vi "oa_Check Tach Pulses Data for Waveform Reference (N Channels).vi"(7 "reset? (True)":bool=TRUE, 8 "error in (no error)":errorcluster, 9 "interpolated pulse positions":dbl[](array[numeric]) format="%.2f", 10 "speed profile":T1 {"speed [RPM]" format="%.2f"; "time [s]" format="%.2f"}, 11 "even angle signals":cluster{"r0":dbl, "dr":dbl, "Y":dbl[]}[](array[cluster]) {"r0" format="%.2p"; "dr" format="%.2p"; "Y" format="%.2f"}) -> (0 "error out":errorcluster, 1 "interpolated pulse positions out":dbl[](array[numeric]) format="%.2f", 2 "speed profile out":T1 {"speed [RPM]" format="%.2f"; "time [s]" format="%.2f"}, 3 "even angle signals":cluster{"r0":dbl, "dr":dbl, "Y":dbl[]}[](array[cluster]) {"r0" format="%.2p"; "dr" format="%.2p"; "Y" format="%.2f"}, 5 "reset":bool)   [LabVIEW 2017]
uses:
  <vilib>/addons/Sound and Vibration/Order Analysis/Tach Process/SubVIs/speed profile.ctl
  <vilib>/addons/Sound and Vibration/Order Analysis/Tach Process/SoundVib_TachProcess.lvlib
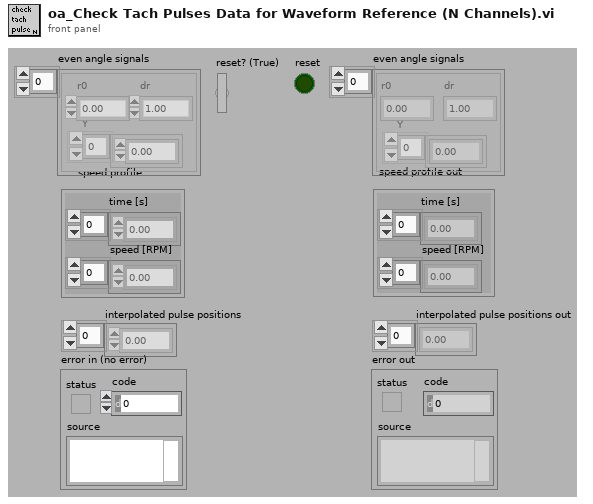
[diagram p1: front panel]
types:
  T1 = typedef "SoundVib_TachProcess.lvlib/speed profile.ctl" = cluster{"time [s]":dbl[], "speed [RPM]":dbl[]}
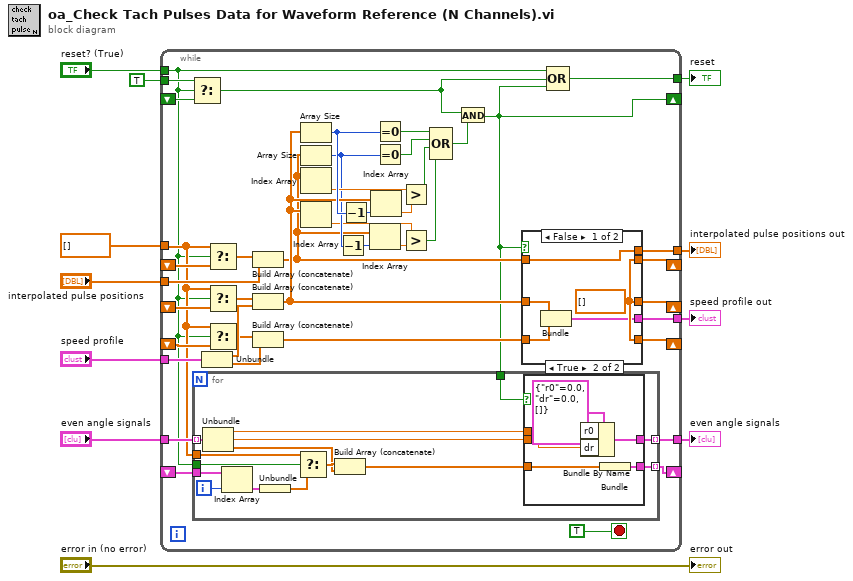
[diagram p0: block diagram]
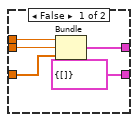
[diagram p2: hidden frame]
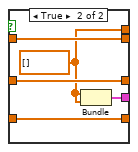
[diagram p3: hidden frame]
diagram:
  n1 = while {
    tunnel: "reset? (True)" -> [w15]
    shift-right: [w13] -> _
    shift-left: _ -> [w53]
    tunnel: "interpolated pulse positions" -> [w48]
    tunnel: "speed profile" -> [w52]
    tunnel: "even angle signals" -> [w51]
    shift-right: [w20] -> _
    shift-left: _ -> [w19]
    tunnel: dbl[] [] ("Y") -> [w18]
    shift-right: [w47] -> _
    shift-left: _ -> [w50]
    tunnel: [w46] -> w4
    shift-right: [w43] -> _
    shift-left: _ -> [w45]
    shift-right: [w38] -> _
    shift-left: _ -> [w40]
    tunnel: [w36] -> w7
    tunnel: TRUE -> [w35]
    tunnel: [w17] -> w2
    tunnel: [w12] -> w1
    stop <- TRUE stop-if-true
    n2 = Select(t=w35, s=w15, f=w53) -> (s? t:f=w14:bool)
    n3 = Unbundle(w52) -> ("time [s]"=w44:dbl[], "speed [RPM]"=w39:dbl[])
    n4 = Select(t=w18, s=w15, f=w50) -> (s? t:f=w49:dbl[])
    n5 = Select(t=w18, s=w15, f=w45) -> (s? t:f=w41:dbl[])
    n6 = Select(t=w18, s=w15, f=w40) -> (s? t:f=w42:dbl[])
    n7 = Build Array (concatenate)(w49, w48) -> (w28:dbl[])
    n8 = Build Array (concatenate)(w41, w44) -> (w31:dbl[])
    n9 = Build Array (concatenate)(w42, w39) -> (w37:dbl[])
    n10 = Array Size(array=w31) -> (size(s)=w34:i32)
    n11 = Array Size(array=w28) -> (size(s)=w29:i32)
    n12 = Index Array(array=w28) -> (element=w33:dbl)  [unwired: 1 in]
    n13 = Index Array(array=w31) -> (element=w25:dbl)  [unwired: 1 in]
    n14 = Decrement(x=w29) -> (x-1=w27:i32)
    n15 = Decrement(x=w34) -> (x-1=w30:i32)
    n16 = Index Array(array=w28, index=w27) -> (element=w26:dbl)
    n17 = Index Array(array=w31, index=w30) -> (element=w32:dbl)
    n18 = Equal To 0?(x=w34) -> (x = 0?=w24:bool)
    n19 = Equal To 0?(x=w29) -> (x = 0?=w23:bool)
    n20 = Greater?(x=w33, y=w32) -> (0:w22:bool)
    n21 = Greater?(x=w25, y=w26) -> (0:w21:bool)
    n22 = Compound Arithmetic op=OR(w24, w23, w22, w21) -> (w16:bool)
    n23 = And(x=w14, y=w16) -> (x .and. y?=w13:bool)
    n24 = for {
      tunnel: w19 -> [w60]
      tunnel: w51 -> [w69] mode=indexing
      tunnel: w15 -> [w67]
      tunnel: w13 -> [w66]
      tunnel: [w62] -> w20 mode=indexing
      tunnel: w18 -> [w61]
      tunnel: [w55] -> w17 mode=indexing
      i -> [w58]
      n25 = Unbundle(w69) -> ("r0"=w65:dbl, "dr"=w64:dbl, "Y"=w59:dbl[])
      n26 = Index Array(array=w60, index=w58) -> (element=w57:cluster{dbl[]})
      n27 = Unbundle(w57) -> (w56:dbl[])
      n28 = Select(t=w61, s=w67, f=w56) -> (s? t:f=w68:dbl[])
      n29 = Build Array (concatenate)(w68, w59) -> (w63:dbl[])
      n30 = case shown="True" w66 {
        tunnel: w65 -> [w74 w77]
        tunnel: w64 -> [w73 w76]
        tunnel: w63 -> [w72 w80]
        tunnel: [cluster{dbl[]} {[]} w79] -> w62
        tunnel: [w71 w75] -> w55
        frame False {
          n31 = Bundle("r0"=w74, "dr"=w73, w72) -> (w71:cluster{"r0":dbl, "dr":dbl, dbl[]})  [unwired: 1 in]
        }
        frame True {
          n32 = Bundle By Name(cluster=cluster{"r0":dbl, "dr":dbl, dbl[]} {"r0"=0.0, "dr"=0.0, []}, "r0"=w77, "dr"=w76) -> (w75:cluster{"r0":dbl, "dr":dbl, dbl[]})
          n33 = Bundle(w80) -> (w79:cluster{dbl[]})  [unwired: 1 in]
        }
      }
    }
    n34 = case shown="False" w13 {
      tunnel: w28 -> [w85 w90]
      tunnel: [w82 w90] -> w47
      tunnel: [w85 w87] -> w46
      tunnel: w31 -> [w84 w89]
      tunnel: [w82 w89] -> w43
      tunnel: [w82 w88] -> w38
      tunnel: w37 -> [w83 w88]
      tunnel: [w81 w86] -> w36
      frame False {
        w82 = dbl[] []
        n35 = Bundle(w84, w83) -> (w81:cluster{dbl[], dbl[]})  [unwired: 1 in]
      }
      frame True {
        w87 = dbl[] []
        n36 = Bundle(w87, w87) -> (w86:cluster{dbl[], dbl[]})  [unwired: 1 in]
      }
    }
    n37 = Compound Arithmetic op=OR(w15, w14, w13) -> (w12:bool)
  }
  "interpolated pulse positions out" <- w4
  "speed profile out" <- w7
  "reset" <- w1
  "even angle signals" <- w2
  "error out" <- "error in (no error)"
